vi "testInitMission.vi"() -> ()   [LabVIEW 2013]
uses:
  Data/TypeDefs/MissionTypeControl.ctl
  Data/TypeDefs/UTM Location.ctl
  Idle/Idle.lvclass
  GoTo/GoTo.lvclass
  RoundBouy/RoundBouy.lvclass
  PassBouy/PassBouy.lvclass
  StationKeeping/StationKeeping.lvclass
  GenericMission.lvclass
  Waypoint/Waypoint.lvclass
panel:
  in  "PoI 2":T1 {"North" format="%#_10f"; "East" format="%#_8f"}
  in  "PoI 1":T1 {"North" format="%#_10f"; "East" format="%#_8f"}
  out "Waypoints out":T1[](array[typedef]) {"North" format="%#_10f"; "East" format="%#_8f"}
  in  "Mission Type":T2
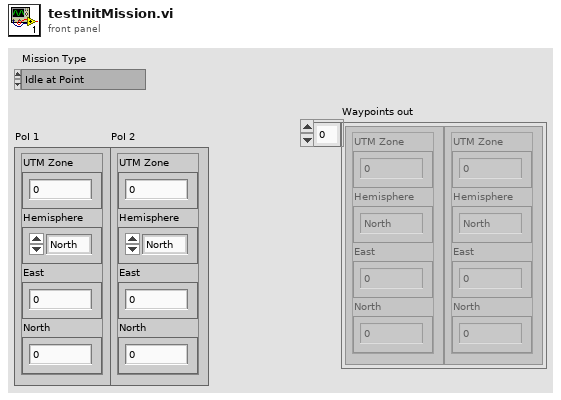
[diagram p1: front panel]
types:
  T1 = typedef "UTM Location.ctl" = cluster{"UTM Zone":dbl, "Hemisphere":enum16{"North", "South"}, "East":dbl, "North":dbl}
  T2 = typedef "MissionTypeControl.ctl" = enum16{"Idle at Point", "Drive to Waypoint", "Round Buoy to Port", "Round Buoy to Starboard", "Pass Between Buoys", "Station Keeping"}
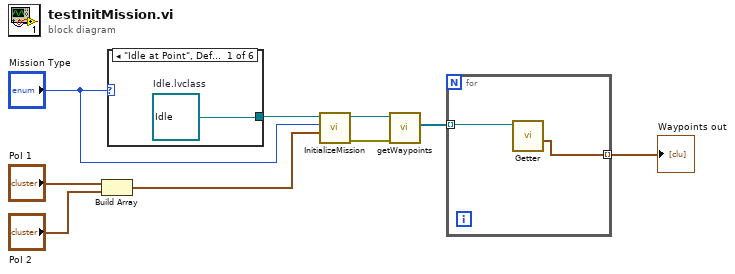
[diagram p0: block diagram]
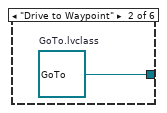
[diagram p2: hidden frame]
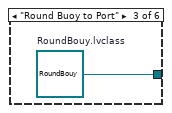
[diagram p3: hidden frame]
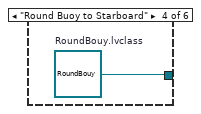
[diagram p4: hidden frame]
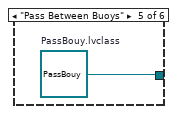
[diagram p5: hidden frame]
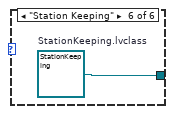
[diagram p6: hidden frame]
diagram:
  n1 = Build Array("PoI 1", "PoI 2") -> (w1:T1[])
  n2 = case shown="\"Idle at Point\", Default" "Mission Type" {
    tunnel: [w10 w11 w12 w13 w14 w15] -> w9
    frame "Idle at Point", Default {
      w10 = refnum<class "Idle.lvclass"> refnum  # Idle.lvclass
    }
    frame "Drive to Waypoint" {
      w11 = refnum<class "GoTo.lvclass"> refnum  # GoTo.lvclass
    }
    frame "Round Buoy to Port" {
      w12 = refnum<class "RoundBouy.lvclass"> refnum  # RoundBouy.lvclass
    }
    frame "Round Buoy to Starboard" {
      w13 = refnum<class "RoundBouy.lvclass"> refnum  # RoundBouy.lvclass
    }
    frame "Pass Between Buoys" {
      w14 = refnum<class "PassBouy.lvclass"> refnum  # PassBouy.lvclass
    }
    frame "Station Keeping" {
      w15 = refnum<class "StationKeeping.lvclass"> refnum  # StationKeeping.lvclass
    }
  }
  n3 = call-dynamic "InitializeMission.vi"("Points of Interest"=w1, "Mission Type"="Mission Type", "GenericMission in"=w9) -> ("Error Out"=w6:errorcluster, "GenericMission out"=w8:refnum<class "GenericMission.lvclass">)  [unwired: 7 in]
  n4 = call-dynamic "getWaypoints.vi"("Error In"=w6, "GenericMission in"=w8) -> ("Waypoint Array"=w5:refnum<class "Waypoint.lvclass">[])  [unwired: 7 in, 2 out]
  n5 = for {
    tunnel: w5 -> [w17] mode=indexing
    tunnel: [w16] -> w4 mode=indexing
    n6 = call "Getter.vi"("Waypoint In"=w17) -> ("Coords"=w16:T1)  [unwired: 6 in, 4 out]
  }
  "Waypoints out" <- w4
